vi "HVBuncher.SetChannelOnOff.vi"(0 "i ref in":refnum<vi>, 1 "ChannelNr":i32, 2 "SetOnOff":bool, 3 "ms timeout (10000)":i32=10000, 5 "error in (no error)":errorcluster) -> (14 "i ref out":refnum<vi>, 17 "timed out":bool, 19 "error out":errorcluster)   [LabVIEW 2014, in "HVBuncher.lvlib"]
doc: "Changes the status (on/off)"
uses:
  HVBuncher.lvlib
  CSCore/CSSystem/CoreDefs/CoreDefs.call_type.ctl
  CSCore/BaseProcess/BaseProcess.descriptor string definition.ctl
  CSCore/CSSystem/CoreDefs/CoreDefs.rawDataType.ctl
  CSCore/CSApplicationBaseClasses/PSChannelBase/PSChannelBase.directionType.ctl
  CSCore/CSApplicationBaseClasses/PSChannelBase/PSChannelBase.serviceType.ctl
  CSCore/CSSystem/CoreLib/CoreLib.short 2 byte array.vi
  CSCore/BaseProcess/BaseProcess.lvlib
  CSCore/CSSystem/CoreLib/CoreLib.lvlib
  CSCore/CSApplicationBaseClasses/DeviceBase/DeviceBase.lvlib
  CSCore/CSApplicationBaseClasses/PSChannelBase/PSChannelBase.lvlib
panel:
  in  "call cluster type":T1={"Object"="", "Selector"="", "CallType"=enum."synchronous", "Async Object"="", "Async Selector"="", "Data Descriptor"="", "Data"=[], "Error #"=0, "Expire"=0}
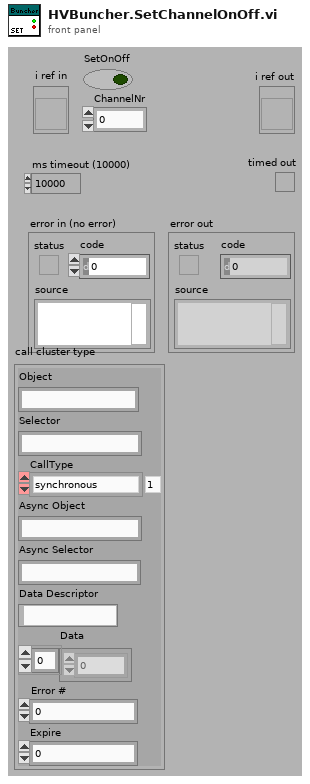
[diagram p1: front panel]
types:
  T1 = typedef "CoreDefs.call_type.ctl" = cluster{"Object":string, "Selector":string, "CallType":enum16{"simple", "synchronous", "asynchronous"}, "Async Object":string, "Async Selector":string, "Data Descriptor":T2, "Data":T3, "Error #":i32, "Expire":u32}
  T2 = typedef "BaseProcess.lvlib/BaseProcess.descriptor string definition.ctl" = string
  T3 = typedef "CoreDefs.rawDataType.ctl" = i8[]
  T4 = typedef "PSChannelBase.lvlib/PSChannelBase.serviceType.ctl" = enum16{"onOff", "voltage", "current", "tripCurrent", "rampUpSpeed", "rampDownSpeed", "status"}
  T5 = typedef "PSChannelBase.lvlib/PSChannelBase.directionType.ctl" = enum16{"unknown", "update actual value", "update nominal value", "update both"}
  T6 = typedef "HVBuncher.lvlib/HVBuncher.i attribute.ctl" = cluster{"ObjectsInitialized":bool, "ChildObjects":T7}
  T7 = typedef "HVBuncher.lvlib/HVBuncher.ChildObjects.ctl" = cluster{"ObjectsLoaded":string[], "actVoltage":dbl[]}
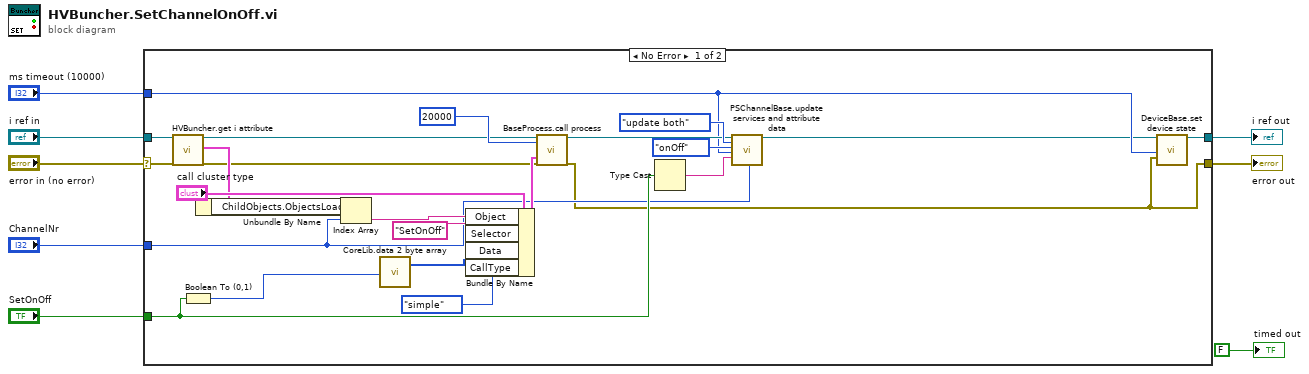
[diagram p0: block diagram]
diagram:
  n1 = case shown="No Error" "error in (no error)" {
    selector: "error in (no error)" -> [w24 w33]
    tunnel: "i ref in" -> [w25 w34]
    tunnel: [w14 w34] -> w7
    tunnel: [w10 w33] -> w5
    tunnel: "ms timeout (10000)" -> [w12 _]
    tunnel: "SetOnOff" -> [w13 _]
    tunnel: "ChannelNr" -> [w11 _]
    frame No Error {
      n2 = call "HVBuncher.get i attribute.vi"("i ref in"=w25, "error in (no error)"=w24) -> ("i ref out"=w20:refnum<vi>, "i attribute"=w23:T6, "error out"=w19:errorcluster)  [unwired: 15 in]
      n3 = Boolean To (0,1)(Boolean=w13) -> (0, 1=w26:i16)
      n4 = Unbundle By Name(w23) -> ("ChildObjects.ObjectsLoaded"=w22:string[])
      n5 = Index Array(array=w22, index=w11) -> (element=w21:string)
      n6 = call-poly "CoreLib.data 2 byte array.vi"("i16"=w26) -> ("byteArray out"=w31:T3)  [unwired: 18 in]
      n7 = Bundle By Name(cluster="call cluster type", "Object"=w21, "Selector"="SetOnOff", "Data"=w31, "CallType"=enum16{"simple", "synchronous", "asynchronous"}."simple") -> (w29:T1)
      n8 = call "BaseProcess.call process.vi"("i ref in"=w20, "timeout (ms)"=20000, "call cluster in"=w29, "error in (no error)"=w19) -> ("i ref out"=w15:refnum<vi>, "error out"=w10:errorcluster)  [unwired: 13 in, 1 out]
      n9 = Type Cast(x=w13) -> (*(type *) &x=w17:string)  [unwired: 1 in]
      n10 = call "PSChannelBase.update services and attribute data.vi"("i ref in"=w15, "direction"=PSChannelBase.directionType."update both", "service"=PSChannelBase.serviceType."onOff", "ms timeout (10000)"=w12, "value"=w17, "channelNumber"=w11) -> ("i ref out"=w9:refnum<vi>)  [unwired: 11 in, 2 out]
      n11 = call "DeviceBase.set device state.vi"("i ref in"=w9, "ms timeout (10000)"=w12, "device error"=w10) -> ("i ref out"=w14:refnum<vi>)  [unwired: 14 in, 2 out]
    }
    frame Error {
    }
  }
  "error out" <- w5
  "i ref out" <- w7
  "timed out" <- FALSE ("timed out")
